vi "Conf Totalizer.vi"(0 "VISA Resource Name":refnum<visa-resource-name>, 1 "Channel List(empty)":string, 5 "Set/Check (F:Set)":bool, 7 "Automatic Reset? (F: No)":bool, 9 "Edge Detect (Falling)":bool, 11 "error in (no error)":errorcluster, 12 "Check Parameter(0:Auto Reset)":enum16{"Automatic Reset", "Edge Detect"}(ring)) -> (4 "VISA Resource Name Out":refnum<visa-resource-name>, 8 "Configuration?":string, 15 "error out":errorcluster)   [LabVIEW 2012, in "Agilent 34970.lvlib"]
doc: "This VI configures the instrument for advanced totalizer readings."
uses:
  <instrlib>/Agilent 34970/Agilent 34970.lvlib
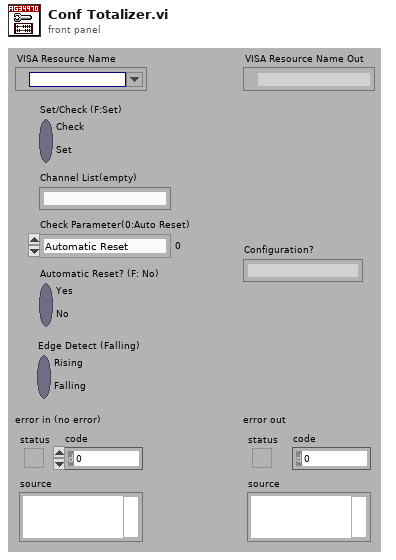
[diagram p1: front panel]
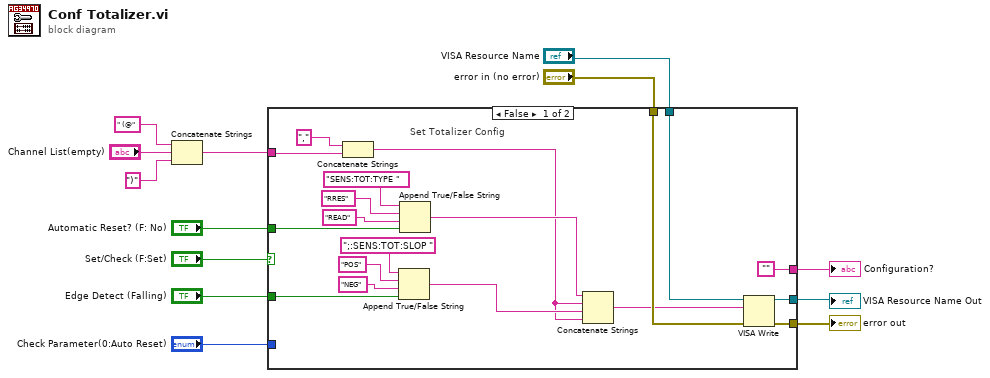
[diagram p0: block diagram]
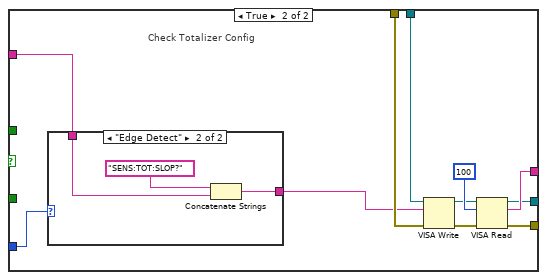
[diagram p2: hidden frame]
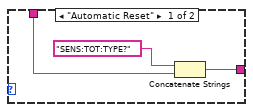
[diagram p3: hidden frame]
diagram:
  n1 = Concatenate Strings(" (@", "Channel List(empty)", ")") -> (w8:string)
  n2 = case shown="False" "Set/Check (F:Set)" {
    tunnel: [w26 w43] -> w1
    tunnel: [w27 w40] -> w2
    tunnel: "Automatic Reset? (F: No)" -> [w24 _]
    tunnel: w8 -> [w32 w34]
    tunnel: ["" w41] -> w7
    tunnel: "VISA Resource Name" -> [w29 w39]
    tunnel: "error in (no error)" -> [w28 w38]
    tunnel: "Check Parameter(0:Auto Reset)" -> [_ w35]
    tunnel: "Edge Detect (Falling)" -> [w20 _]
    frame False {
      # "Set Totalizer Config"
      n3 = Concatenate Strings(",", w32) -> (w16:string)
      n4 = Append True/False String(1:w20, 2:"NEG" ("false string"), 3:"POS" ("true string"), 4:";:SENS:TOT:SLOP ") -> (0:w18:string)
      n5 = Append True/False String(1:w24, 2:"READ" ("false string"), 3:"RRES" ("true string"), 4:"SENS:TOT:TYPE ") -> (0:w19:string)
      n6 = Concatenate Strings(w19, w16, w18, w16) -> (w17:string)
      n7 = VISA Write(VISA resource name=w29, write buffer=w17, error in (no error)=w28) -> (VISA resource name out=w27:refnum<visa-resource-name>, error out=w26:errorcluster)  [unwired: 1 out]
    }
    frame True {
      # "Check Totalizer Config"
      n8 = case shown="\"Edge Detect\"" w35 {
        tunnel: w34 -> [w45 w48]
        tunnel: [w46 w49] -> w33
        frame "Automatic Reset" {
          n9 = Concatenate Strings("SENS:TOT:TYPE?", w45) -> (w46:string)
        }
        frame "Edge Detect" {
          n10 = Concatenate Strings("SENS:TOT:SLOP?", w48) -> (w49:string)
        }
      }
      n11 = VISA Write(VISA resource name=w39, write buffer=w33, error in (no error)=w38) -> (VISA resource name out=w37:refnum<visa-resource-name>, error out=w36:errorcluster)  [unwired: 1 out]
      n12 = VISA Read(VISA resource name=w37, byte count=u32 100 ("byte count (0)"), error in (no error)=w36) -> (VISA resource name out=w40:refnum<visa-resource-name>, read buffer=w41:string, error out=w43:errorcluster)  [unwired: 1 out]
    }
  }
  "Configuration?" <- w7
  "error out" <- w1
  "VISA Resource Name Out" <- w2
